vi "gfitsio-windows-message-box.vi"(4 "enable dialog?":bool, 5 "Modality (Application)":u32(ring) items=["Application"=0, "System"=4096, "Task"=8192, "Help"=16384], 6 "Icon (None)":u32(ring) items=["None"=0, "Warning"=48, "Confirmation"=64, "Question"=32, "Error"=16, "User Icon"=128], 7 "Default (Button 1)":u32(ring) items=["Button 1"=0, "Button 2"=256, "Button 3"=512, "Button 4"=1024], 8 "Buttons (OK)":u32(ring) items=["Abort/Retry/Ignore"=2, "OK"=0, "OK/Cancel"=1, "Retry/Cancel"=5, "Yes/No"=4, "Yes/No/Cancel"=3], 10 "Text":string, 11 "Title":string) -> (3 "Button Selected":T1(ring))   [LabVIEW 2023, in "gfitsio.lvlib"]
doc: "The MessageBox function creates, displays, and operates a message box. The message box contains an application-defined message and title, along with any combination of predefined icons and push buttons.\n\nIf a message box has a Cancel button, the function returns the IDCANCEL value if either the ESC key is pressed or the Cancel button is selected. If the message box has no Cancel button, pressing ESC has no effect."
uses:
  gfitsio.lvlib
  gfitsio.dll
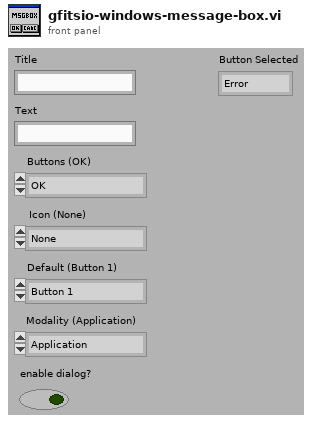
[diagram p1: front panel]
types:
  T1 = enum16{"Error", "Ok", "Cancel", "Abort", "Retry", "Ignore", "Yes", "No", "Close", "Help", "Disabled"}
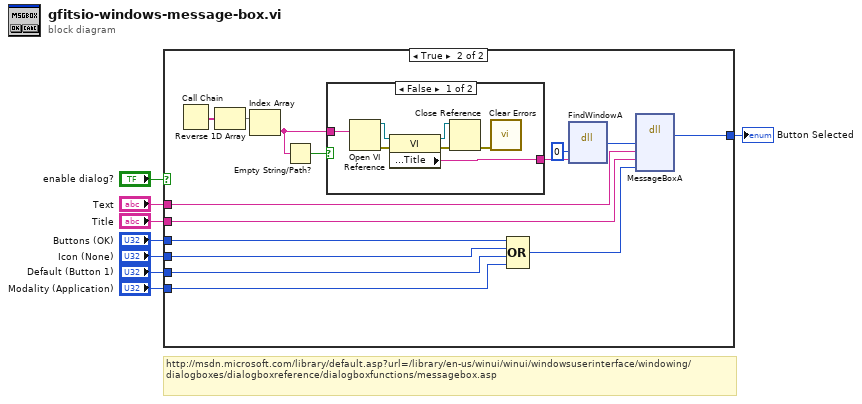
[diagram p0: block diagram]
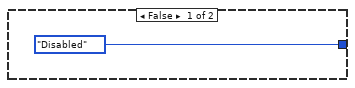
[diagram p2: hidden frame]
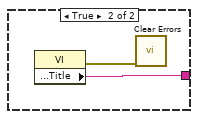
[diagram p3: hidden frame]
diagram:
  # "http://msdn.microsoft.com/library/default.asp?url=/library/en-us/winui/winui/windowsuserinterface/windowing/dialogboxes/dialogboxreference/dialogboxfunctions/messagebox.asp"
  n1 = case shown="True" "enable dialog?" {
    tunnel: "Text" -> [_ w20]
    tunnel: "Title" -> [_ w19]
    tunnel: [T1."Disabled" ("Button Selected") w18] -> w6
    tunnel: "Buttons (OK)" -> [_ w15]
    tunnel: "Icon (None)" -> [_ w14]
    tunnel: "Default (Button 1)" -> [_ w13]
    tunnel: "Modality (Application)" -> [_ w12]
    frame False {
    }
    frame True {
      n2 = Call Chain() -> (call chain=w11:string[])
      n3 = Reverse 1D Array(array=w11) -> (reversed array=w10:string[])
      n4 = Index Array(array=w10) -> (element=w16:string)  [unwired: 1 in]
      n5 = Empty String/Path?(string/path=w16) -> (empty?=w17:bool)
      n6 = case shown="False" w17 {
        tunnel: [w31 w33] -> w24
        tunnel: w16 -> [w26 _]
        frame False {
          n7 = Open VI Reference(vi path=w26) -> (vi reference=w29:refnum<vi>, error out=w30:errorcluster)  [unwired: 1 in, 4 out]
          n8 = property class="VI"(reference=w29, error in=w30) -> (reference out=w27:refnum<vi>, error out=w28:errorcluster, "Front Panel Window:Title"=w31:string)
          n9 = Close Reference(reference=w27, error in (no error)=w28) -> (error out=w25:errorcluster)
          n10 = call <vilib>:"Clear Errors.vi"("error in (no error)"=w25) -> ()  [unwired: 1 in, 6 out]
        }
        frame True {
          n11 = property class="VI"() -> (error out=w32:errorcluster, "Front Panel Window:Title"=w33:string)  [unwired: 2 in, 1 out]
          n12 = call <vilib>:"Clear Errors.vi"("error in (no error)"=w32) -> ()  [unwired: 1 in, 6 out]
        }
      }
      n13 = Compound Arithmetic op=OR(w15, w14, w13, w12) -> (w22:u32)
      n14 = dll-call lib="gfitsio.dll" fn="FindWindowA" label="FindWindow"("lpszClassName"=0, "lpszWindowName"=w24) -> ("hWnd"=w23:u32)  [unwired: 5 in, 2 out]
      n15 = dll-call lib="gfitsio.dll" fn="MessageBoxA"("hWnd"=w23, "lpText"=w20, "lpCaption"=w19, "uType"=w22) -> (w18:i32)  [unwired: 7 in, 2 out]
    }
  }
  "Button Selected" <- w6
